vi "RepeatString.vi"(10 "NumTimes":i32, 11 "String [in]":string) -> (3 "RepeatedString [out]":string)   [LabVIEW 2012]
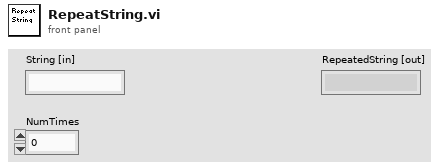
[diagram p1: front panel]
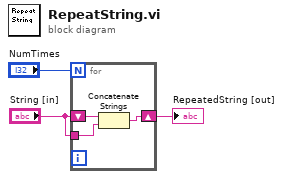
[diagram p0: block diagram]
diagram:
  n1 = for {
    N: "NumTimes" -> [_]
    shift-right: [w4] -> w1
    shift-left: "String [in]" -> [w6]
    tunnel: "String [in]" -> [w5]
    n2 = Concatenate Strings(w6, w5) -> (w4:string)
  }
  "RepeatedString [out]" <- w1
